vi "Write Popup ViewManager Type.vi"(6 "Popup ViewManager Type":refnum<class "Popup ViewManager.lvclass">, 11 "Main View in":refnum<class "Main View.lvclass">) -> (3 "Main View out":refnum<class "Main View.lvclass">)   [LabVIEW 2017, in "Main View.lvclass"]
uses:
  <vilib>/gpm_packages/@cs/popup-viewmanager/Example/Main View/Main View.lvclass
  <vilib>/gpm_packages/@cs/popup-viewmanager/Source/Popup ViewManager/Popup ViewManager.lvclass
  <vilib>/gpm_packages/@cs/popup-viewmanager/Example/Main View/Main View.lvclass/Main View.ctl
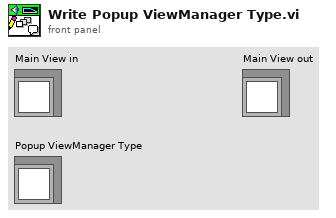
[diagram p1: front panel]
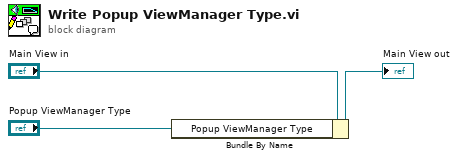
[diagram p0: block diagram]
diagram:
  n1 = Bundle By Name(cluster="Main View in", "Popup ViewManager Type"="Popup ViewManager Type") -> (→"Main View out":refnum<class "Main View.lvclass">)
